vi "Light Level Read.vi"() -> (0 "Brightness":i32, 1 "Exposure":i32, 2 "Input Voltage (A3)":dbl)   [LabVIEW 2013]
uses:
  <vilib>/myRIO/Instrument Drivers/Onboard IO/AI/vis/Smart Open.vi
  <vilib>/myRIO/Instrument Drivers/Onboard IO/AI/vis/Read.vi
  <vilib>/myRIO/Instrument Drivers/Onboard IO/AI/vis/Open.vi
  <vilib>/myRIO/Common/Instrument Driver Framework/myRIO v1.0/AI/vis/myRIO v1.1 Open AI.vi
  <vilib>/myRIO/Common/Instrument Driver Framework/Utilities/vis/Validate Channels.vi
  <vilib>/myRIO/Common/Instrument Driver Framework/myRIO v1.0/AI/vis/myRIO v1.0 Reserve AI.vi
  <vilib>/myRIO/Common/Instrument Driver Framework/myRIO v1.0/AI/vis/myRIO v1.0 Build MUX Configuration AI.vi
  <vilib>/myRIO/Common/Instrument Driver Framework/myRIO v1.0/Resource Manager/vis/myRIO v1.0 Reserve Channel List.vi
  <vilib>/myRIO/Common/Instrument Driver Framework/myRIO v1.0/Resource Manager/vis/myRIO v1.0 Reserve Channel.vi
  <vilib>/myRIO/Common/Instrument Driver Framework/myRIO v1.0/Resource Manager/vis/myRIO v1.0 Unreserve Channel.vi
  <vilib>/myRIO/Common/Instrument Driver Framework/myRIO v1.0/Resource Manager/vis/myRIO v1.0 Build Mutex Name.vi
  <vilib>/myRIO/Common/Instrument Driver Framework/myRIO v1.0/myRIO v1.1 Open.vi
  <vilib>/myRIO/Common/Instrument Driver Framework/myRIO v1.0/AI/vis/myRIO v1.0 Get Scaling Constants AI.vi
  <vilib>/Utility/VariantDataType/GetNumericInfo.vi
  <vilib>/Utility/error.llb/Error Cluster From Error Code.vi
  <vilib>/myRIO/Common/Instrument Driver Framework/Utilities/vis/IO Manager.vi
  <vilib>/myRIO/Common/Instrument Driver Framework/Utilities/vis/Configuration Manager.vi
  <vilib>/myRIO/Common/Instrument Driver Framework/myRIO v1.0/myRIO v1.0 Close.vi
  <vilib>/myRIO/Common/Instrument Driver Framework/myRIO v1.0/AI/vis/myRIO v1.0 Read AI.vi
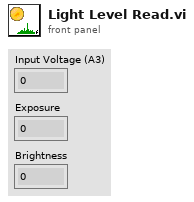
[diagram p1: front panel]
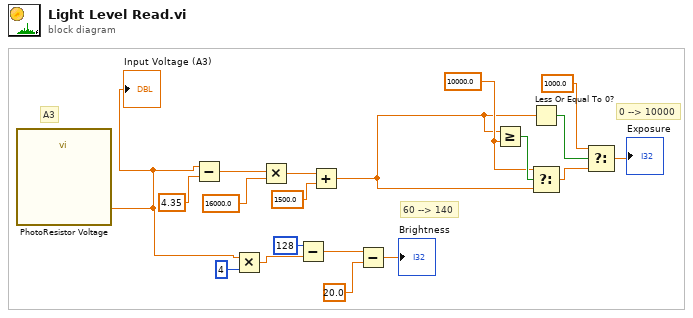
[diagram p0: block diagram]
diagram:
  w3 = 10000.0 ("t")
  # "60 --> 140"
  # "0 --> 10000"
  # "A3"
  n1 = call "PhotoResistor Voltage"() -> ("A/AI0 (Pin 3)"=w1:dbl)  [unwired: 26 in, 1 out]
  "Input Voltage (A3)" <- w1
  n2 = Subtract(x=w1, y=4.35) -> (x-y=w10:dbl)
  n3 = Multiply(x=w1, y=4) -> (x*y=w17:dbl)
  n4 = Multiply(x=w10, y=16000.0) -> (x*y=w11:dbl)
  n5 = Subtract(x=128, y=w17) -> (x-y=w13:dbl)
  n6 = Add(x=w11, y=1500.0) -> (x+y=w2:dbl)
  n7 = Subtract(x=w13, y=20.0) -> (x-y=→"Brightness":dbl)
  n8 = Greater Or Equal?(x=w2, y=w3) -> (x >= y?=w4:bool)
  n9 = Less Or Equal To 0?(x=w2) -> (x <= 0?=w7:bool)
  n10 = Select(t=w3, s=w4, f=w2) -> (s? t:f=w8:dbl)
  n11 = Select(t=1000.0, s=w7, f=w8) -> (s? t:f=→"Exposure":dbl)
